vi "Resize Panel to Pane.vi"(8 "error in (no error)":errorcluster, 10 "Apply Recursively? (F)":bool, 11 "RandomDataChart In":refnum<class "BasicChartBinding.lvclass">) -> (0 "error out":errorcluster, 3 "RandomDataChart Out":refnum<class "BasicChartBinding.lvclass">)   [LabVIEW 2017, in "Integration Test Launcher.lvlib" / "TestViewables.lvlib" / "BasicChartBinding.lvclass"]
doc: "<License>\nCopyright © 2020 Tymphany, LLC | All rights reserved\nwww.Tymphany.com\nHuijun <Huijun.Guo@Tymphany.com>\n</License>"
uses:
  <vilib>/gpm_packages/@cs/example/Integration Test/BasicChartBinding/BasicChartBinding.lvclass
  <vilib>/gpm_packages/@cs/example/Integration Test/BasicChartBinding/BasicChartBinding.lvclass/BasicChartBinding.ctl
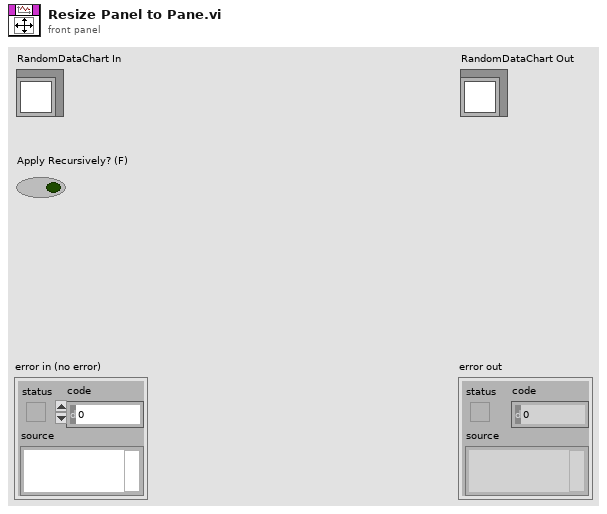
[diagram p1: front panel]
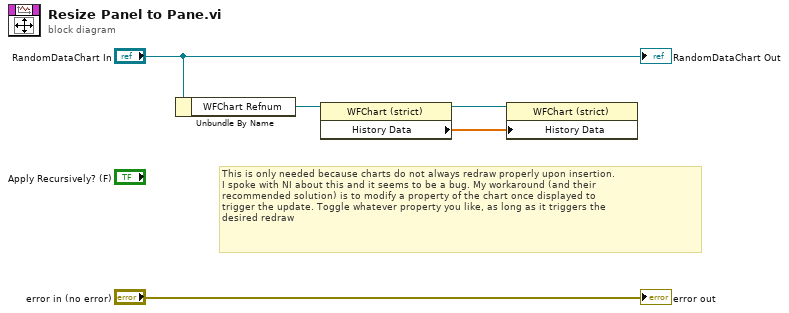
[diagram p0: block diagram]
diagram:
  # "This is only needed because charts do not always redraw properly upon insertion.\nI spoke with NI about this and it seems to be a bug. My workaround (and their\nrecommended solution) is to modify a property of the chart once displayed to\ntrigger the update. Toggle whatever property you like, as long as it triggers the\ndesired redraw"
  n1 = Unbundle By Name("RandomDataChart In") -> ("WFChart Refnum"=w3:refnum<vi>)
  n2 = property class="WFChart (strict)"(reference=w3) -> (reference out=w2:refnum<vi>, "History Data"=w1:dbl[])  [unwired: 1 in, 1 out]
  n3 = property class="WFChart (strict)"(reference=w2, "History Data"=w1) -> ()  [unwired: 1 in, 2 out]
  "error out" <- "error in (no error)"
  "RandomDataChart Out" <- "RandomDataChart In"
